vi "Periodic Tasks.vi"(8 "error in":errorcluster) -> ()   [LabVIEW 2018]
doc: "This VI runs in parallel to other robot code. It can contain as many user-defined periodic loops as you need. These can carry out PID or other sorts of timed response."
uses:
  <vilib>/Rock Robotics/Network Tables/NT Write Number.vi
  Robot Global Data.vi
  <vilib>/Rock Robotics/WPI/ThirdParty/Sensors/ADIS16448 IMU/ADIS16448_IMU.lvlib
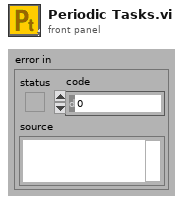
[diagram p1: front panel]
types:
  T1 = typedef "WPI_JoystickDevRef.ctl" = cluster{"Device":T2}
  T2 = typedef "WPI_JoystickDeviceEnum.ctl" = enum16{"USB 0", "USB 1", "USB 2", "USB 3", "USB 4", "USB 5"}
  T3 = typedef "ADIS16448_IMU.lvlib/ADI_IMU_ADIS16448_IMUDevRef.ctl" = cluster{"DevStatus":errorcluster, "Handle":i32, "SPI Bus":T4, "Device Found":bool, "Device Ready":bool, "Yaw Axis":enum16{"X", "Y", "Z"}, "AHRS Algorithm":enum16{"Complementary", "Madgwick"}, "Serial":u16, "Lot ID 2":u16, "Lot ID 1":u16, "Bytes Per Sample":u16, "Calibrate On Open?":bool}
  T4 = typedef "spi_bus.ctl" = enum16{"SPI On-Board, CS0", "SPI On-Board, CS1", "SPI On-Board, CS2", "SPI On-Board, CS3", "SPI MXP", "Invalid"}
  T5 = cluster{"X Angle":dbl, "Y Angle":dbl, "Z Angle":dbl}
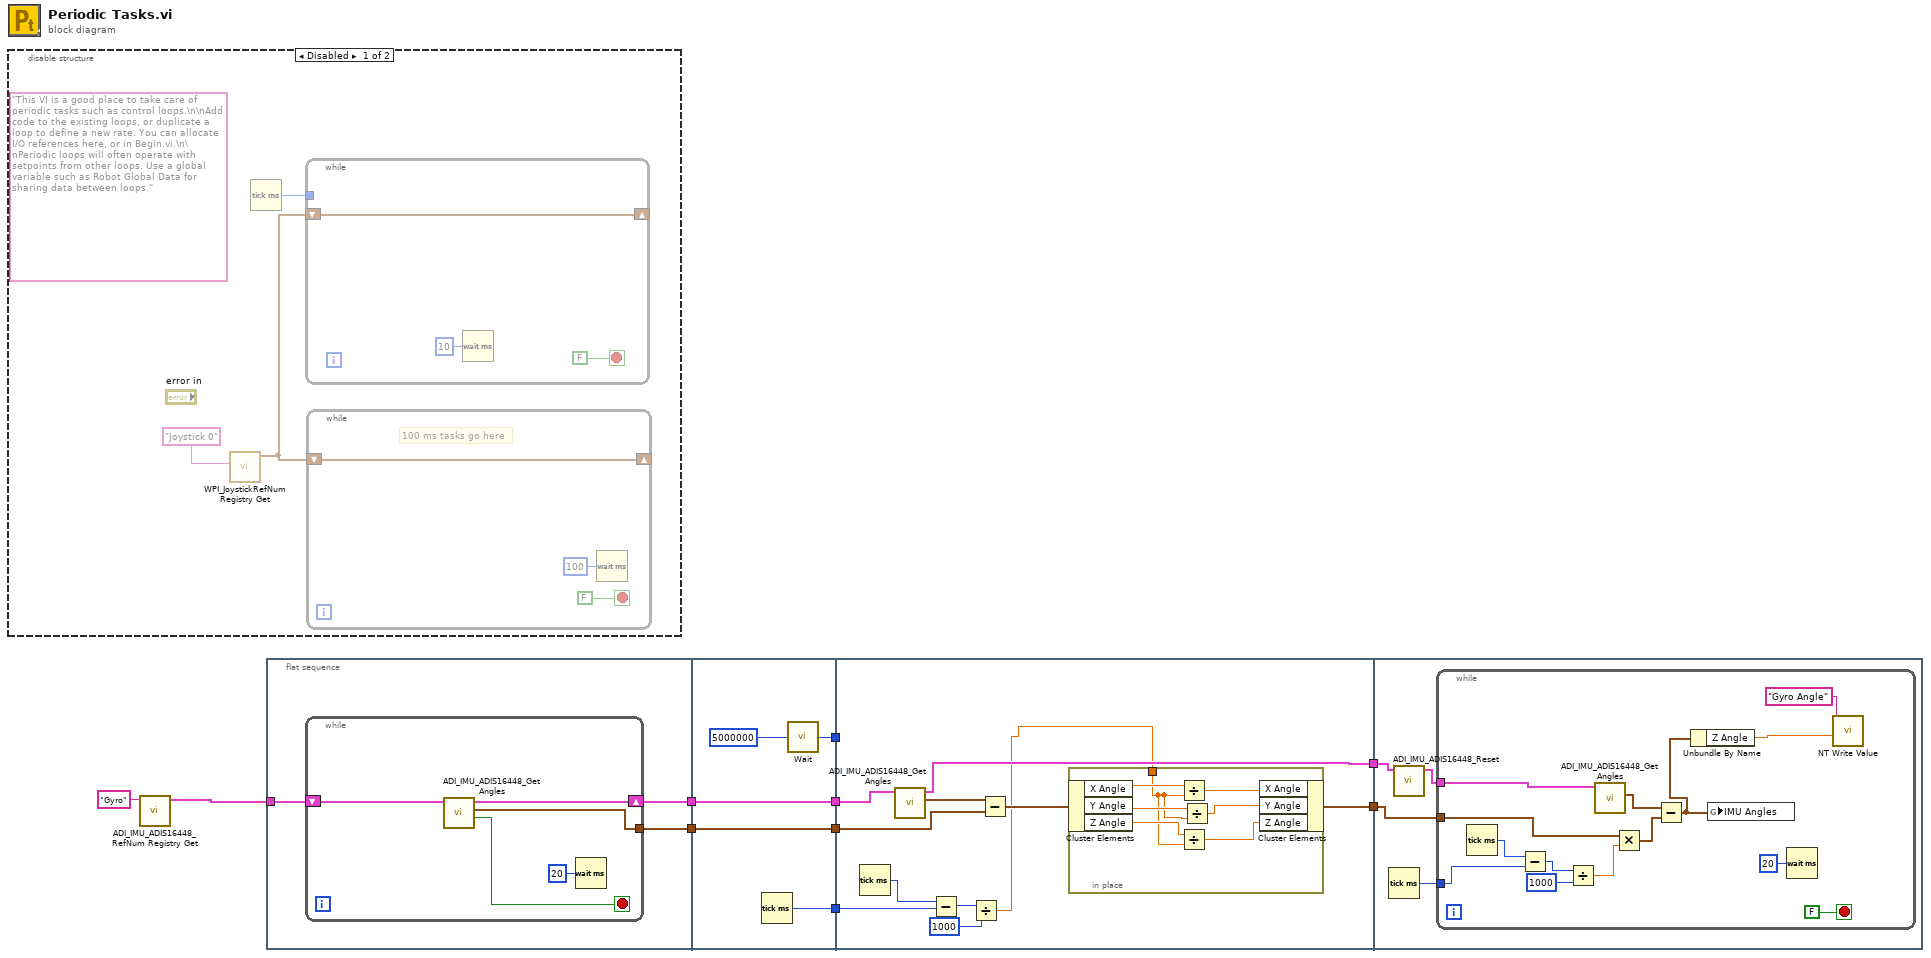
[diagram p0: block diagram]
diagram:
  n1 = disable-structure shown="Disabled" {
    frame Disabled {
      (unwired) "This VI is a good place to take care of periodic tasks such as control loops.\n\nAdd code to the existing loops, or duplicate a loop to define a new rate. You can allocate I/O references here, or in Begin.vi.\n\nPeriodic loops will often operate with setpoints from other loops. Use a global variable such as Robot Global Data for sharing data between loops."
      n2 = call <vilib>:"WPI_JoystickRefNum Registry Get.vi"("refnum name"="Joystick 0") -> ("JoystickDevRef"=w12:T1)  [unwired: 1 in, 9 out]
      n3 = Tick Count (ms)() -> (millisecond timer value=w11:u32)
      n4 = while {
        shift-right: [w18] -> _
        shift-left: w12 -> [w18]
        tunnel: w11 -> [_]
        stop <- FALSE stop-if-true
        n5 = Wait (ms)(milliseconds to wait=u32 10) -> ()  [unwired: 1 out]
      }
      n6 = while {
        shift-right: [w14] -> _
        shift-left: w12 -> [w14]
        stop <- FALSE stop-if-true
        # "100 ms tasks go here"
        n7 = Wait (ms)(milliseconds to wait=u32 100) -> ()  [unwired: 1 out]
      }
    }
    frame Enabled {
    }
  }
  n8 = call <vilib>:"ADI_IMU_ADIS16448_RefNum Registry Get.vi"("refnum name"="Gyro") -> ("ADI IMU DevRef"=w10:T3)  [unwired: 9 in, 1 out]
  n9 = flat-sequence {
    tunnel: w10 -> [w22]
    tunnel: [w21] -> w7
    tunnel: [w20] -> w5
    tunnel: [w31] -> w9
    tunnel: [w30] -> w8
    tunnel: w7 -> [w30]
    tunnel: [w29] -> w6
    tunnel: w5 -> [w29]
    tunnel: [w28] -> w1
    tunnel: w9 -> [_]
    tunnel: w8 -> [w43]
    tunnel: w6 -> [w41]
    tunnel: [w39] -> w4
    tunnel: [w38] -> w3
    tunnel: w1 -> [w37]
    tunnel: w4 -> [w53]
    tunnel: w3 -> [w52]
    frame #0 {
      n10 = while {
        shift-right: [w25] -> w21
        shift-left: w22 -> [w26]
        tunnel: [w23] -> w20
        stop <- w24 stop-if-true
        n11 = call <vilib>:"ADI_IMU_ADIS16448_Get Angles.vi"("ADI IMU DevRef"=w26) -> ("Sensor Ready Out"=w24:bool, "IMU Angles Out"=w23:T5, "ADI IMU DevRef Out"=w25:T3)  [unwired: 7 in, 1 out]
        n12 = Wait (ms)(milliseconds to wait=u32 20) -> ()  [unwired: 1 out]
      }
    }
    frame #1 {
      n13 = Tick Count (ms)() -> (millisecond timer value=w28:u32)
      n14 = call "Wait"("Count(uSec)"=u32 5000000) -> ("Tick Count(uSec)"=w31:u32)
    }
    frame #2 {
      n15 = Tick Count (ms)() -> (millisecond timer value=w36:u32)
      n16 = call <vilib>:"ADI_IMU_ADIS16448_Get Angles.vi"("ADI IMU DevRef"=w43) -> ("IMU Angles Out"=w42:T5, "ADI IMU DevRef Out"=w38:T3)  [unwired: 7 in, 2 out]
      n17 = Subtract(x=w36, y=w37) -> (x-y=w35:u32)
      n18 = Divide(x=w35, y=u32 1000) -> (x/y=w33:dbl)
      n19 = Subtract(x=w42, y=w41) -> (x-y=w40:T5)
      n20 = in-place {
        in-place-border: w33 -> [w44]
        n21 = in-place-cluster #1(w40) -> ("X Angle"=w49:dbl, "Y Angle"=w48:dbl, "Z Angle"=w45:dbl)
        n22 = Divide(x=w49, y=w44) -> (x/y=w50:dbl)
        n23 = Divide(x=w45, y=w44) -> (x/y=w46:dbl)
        n24 = Divide(x=w48, y=w44) -> (x/y=w47:dbl)
        n25 = in-place-cluster #1("X Angle"=w50, "Y Angle"=w47, "Z Angle"=w46) -> (w39:T5)
      }
    }
    frame #3 {
      n26 = Tick Count (ms)() -> (millisecond timer value=w54:u32)
      n27 = call <vilib>:"ADI_IMU_ADIS16448_Reset.vi"("ADI IMU DevRef"=w52) -> ("ADI IMU DevRef Out"=w51:T3)  [unwired: 9 in, 1 out]
      n28 = while {
        tunnel: w54 -> [w67]
        tunnel: w53 -> [w64]
        tunnel: w51 -> [w62]
        stop <- FALSE stop-if-true
        n29 = Tick Count (ms)() -> (millisecond timer value=w68:u32)
        n30 = Subtract(x=w68, y=w67) -> (x-y=w66:u32)
        n31 = Divide(x=w66, y=u32 1000) -> (x/y=w63:dbl)
        n32 = call <vilib>:"ADI_IMU_ADIS16448_Get Angles.vi"("ADI IMU DevRef"=w62) -> ("IMU Angles Out"=w60:T5)  [unwired: 7 in, 3 out]
        n33 = Multiply(x=w64, y=w63) -> (x*y=w61:T5)
        n34 = Subtract(x=w60, y=w61) -> (x-y=w57:T5)
        n35 = Unbundle By Name(w57) -> ("Z Angle"=w56:dbl)
        n36 = global write "Robot Global Data.vi" "IMU Angles"(w57) -> ()
        n37 = Wait (ms)(milliseconds to wait=u32 20) -> ()  [unwired: 1 out]
        n38 = call-poly <vilib>:"NT Write Value.vi"("Numeric"=w56, "Name"="Gyro Angle") -> ()  [unwired: 9 in, 1 out]
      }
    }
  }
